vi "Initialize Range Controller.vi"(6 "Main Controls":refnum<vi>, 8 "error in (no error)":errorcluster, 9 "Ranges Refnum":T1, 10 "Settings":T2, 11 "Range Controller Actor in":refnum<class "Range Controller Actor.lvclass">) -> (0 "error out":errorcluster, 3 "Range Controller Actor out":refnum<class "Range Controller Actor.lvclass">)   [LabVIEW 2018, in "Range Controller.lvlib" / "Range Controller Actor.lvclass"]
uses:
  Range Controller Actor.lvclass
  C:/Program Files (x86)/National Instruments/LabVIEW 2018/vi.lib/ActorFramework/Actor/Actor.lvclass
  MWWL Verification/Type Defs/ConfigSettings.ctl
  MWWL Verification/MWWL Verification/Ranges Refnum.ctl
  Reference Range Actor/Reference Range/Reference Range Actor.lvclass
  Range Controller Actor.lvclass/Range Controller Actor.ctl
  Reference Range Actor/Reference Range Actor Messages/Initialize Reference Range Cart Msg/Initialize Reference Range Cart Msg.lvclass/Initialize Reference Range Cart Msg.ctl
  <vilib>/ActorFramework/Message Enqueuer/Message Enqueuer.lvclass/Message Enqueuer.ctl
  <vilib>/ActorFramework/Message Enqueuer/Enqueue.vi
  Reference Range Actor/Reference Range Actor Messages/Initialize Reference Range Cart Msg/Initialize Reference Range Cart Msg.lvclass
  C:/Program Files (x86)/National Instruments/LabVIEW 2018/vi.lib/ActorFramework/Message/Message.lvclass
  <vilib>/ActorFramework/Message Priority Queue/Priority Enqueue.vi
  <vilib>/ActorFramework/Actor/Actor.lvclass
  MWWL Verification/MWWL Verification.lvlib
panel:
  # "RANGES (m)"
  # "SM140"
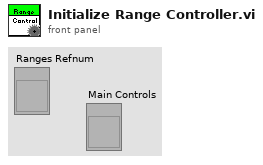
[diagram p1: front panel]
types:
  T1 = typedef "MWWL Verification.lvlib/Ranges Refnum.ctl" = refnum<vi>
  T2 = typedef "MWWL Verification.lvlib/ConfigSettings.ctl" = cluster{"Base Path":path, "DNL_Configuration Settings.Ports":cluster{"Ref. Range COM Port":refnum<visa-resource-name>, "MWWL COM Port":refnum<visa-resource-name>, "ULS COM Port":refnum<visa-resource-name>, "Laser A COM Port":refnum<visa-resource-name>, "Laser B COM Port":refnum<visa-resource-name>, "Laser C COM Port":refnum<visa-resource-name>, "Laser D COM Port":refnum<visa-resource-name>, "AirMar COM Port":refnum<visa-resource-name>}, "H3611i":bool}
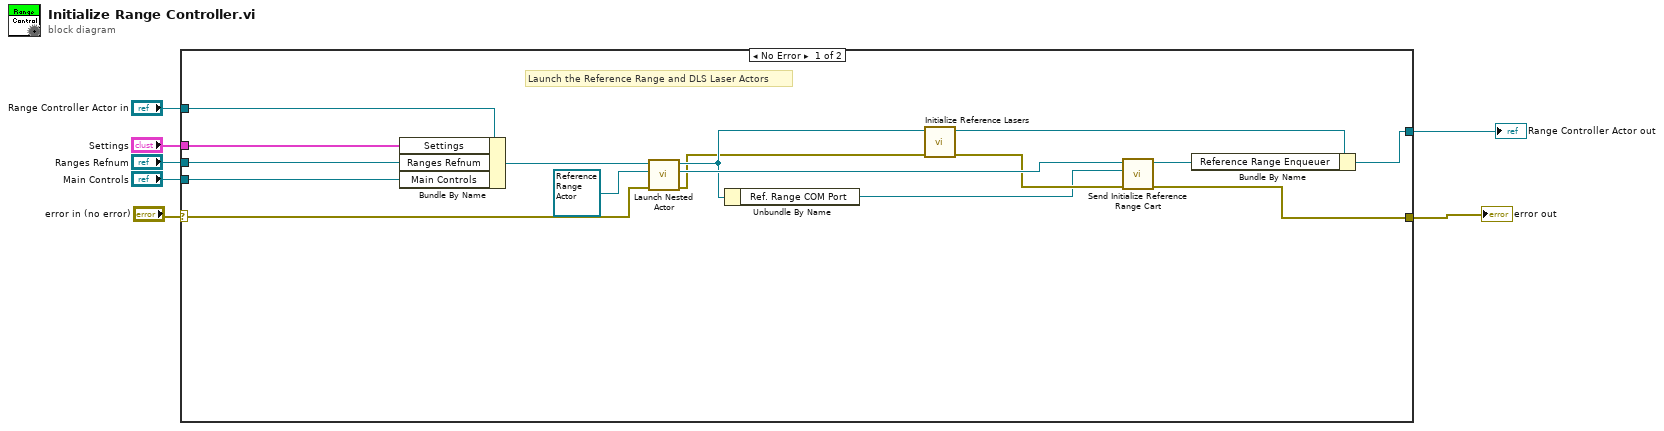
[diagram p0: block diagram]
diagram:
  n1 = case shown="No Error" "error in (no error)" {
    selector: "error in (no error)" -> [w16 w25]
    tunnel: [w15 w25] -> w6
    tunnel: [w20 w24] -> w4
    tunnel: "Range Controller Actor in" -> [w23 w24]
    tunnel: "Settings" -> [w22 _]
    tunnel: "Ranges Refnum" -> [w14 _]
    tunnel: "Main Controls" -> [w8 _]
    frame No Error {
      # "Launch the Reference Range and DLS Laser Actors"
      n2 = Bundle By Name(cluster=w23, "Settings"=w22, "Ranges Refnum"=w14, "Main Controls"=w8) -> (w21:refnum<class "Range Controller Actor.lvclass">)
      n3 = call <vilib>:"Launch Nested Actor.vi"("error in (no error)"=w16, "Nested Actor"=refnum<class "Reference Range Actor.lvclass"> refnum ("Reference Range.lvlib:Reference Range Actor"), "Caller Actor in"=w21) -> ("error out"=w11:errorcluster, "Nested Actor's Enqueuer"=w19:refnum<class "Message Enqueuer.lvclass">, "Caller Actor out"=w13:refnum<class "Range Controller Actor.lvclass">)  [unwired: 6 in]
      n4 = Unbundle By Name(w13) -> ("Ref. Range COM Port"=w9:refnum<visa-resource-name>)
      n5 = call "Initialize Reference Lasers.vi"("error in (no error)"=w11, "Range Controller Actor in"=w13) -> ("error out"=w10:errorcluster, "Range Controller Actor out"=w12:refnum<class "Range Controller Actor.lvclass">)  [unwired: 8 in]
      n6 = call "Send Initialize Reference Range Cart.vi"("error in (no error)"=w10, "Reference Range COM Port"=w9, "Message Enqueuer in"=w19) -> ("error out"=w15:errorcluster, "Message Enqueuer out"=w18:refnum<class "Message Enqueuer.lvclass">)  [unwired: 7 in]
      n7 = Bundle By Name(cluster=w12, "Reference Range Enqueuer"=w18) -> (w20:refnum<class "Range Controller Actor.lvclass">)
    }
    frame Error {
    }
  }
  "error out" <- w6
  "Range Controller Actor out" <- w4
